vi "Test Serialize.vi"() -> ()   [LabVIEW 2016]
uses:
  typedefs/Request--Cluster.ctl
  JSON-RPC.lvclass
  <vilib>/addons/_JKI.lib/Serialization/JSON/JKI JSON Serialization.lvlib
panel:
  in  "Enum":T1(ring)
  out "x = y?":bool
  in  "Numeric":i32=100 format="%.0p"
  out "x-y":dbl format="%#_6p"
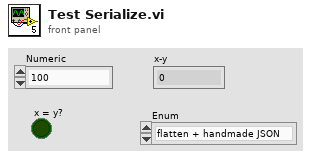
[diagram p1: front panel]
types:
  T1 = enum16{"flatten + handmade JSON", "flatten + JKI JSON", "flatten"}
  T2 = cluster{"jsonrpc":string, "result":string, "error":variant, "id":string}
  T3 = typedef "JSON-RPC.lvclass/Request--Cluster.ctl" = cluster{"method":string, "params":variant, "Notification?":bool}
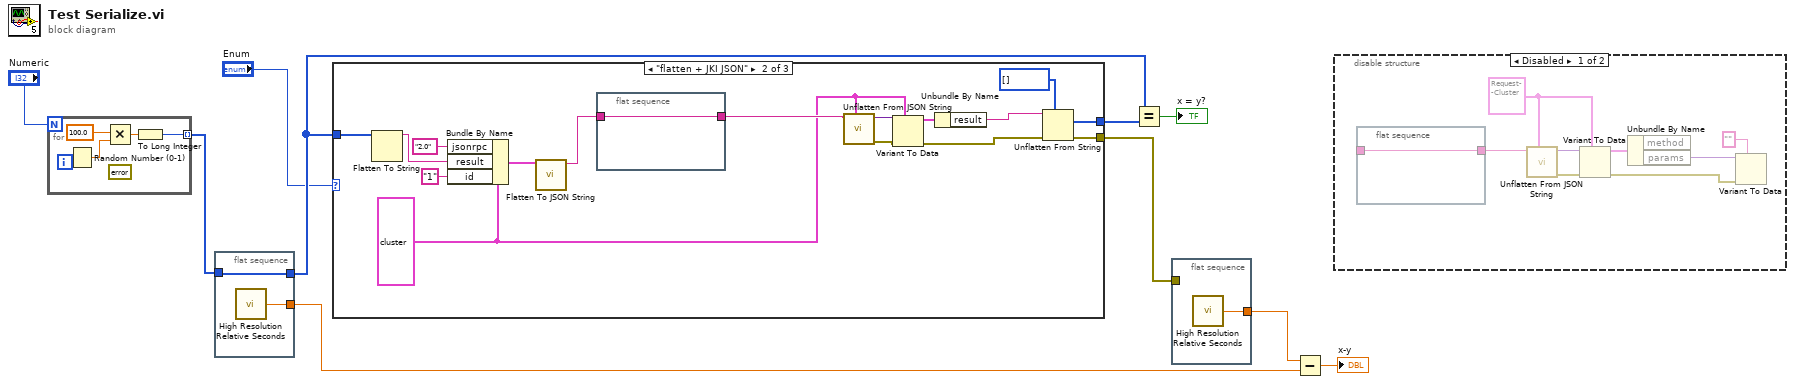
[diagram p0: block diagram]
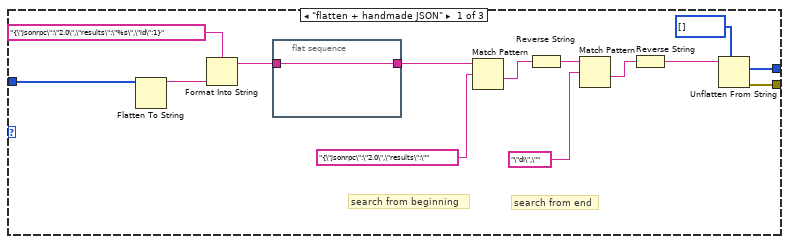
[diagram p2: hidden frame]
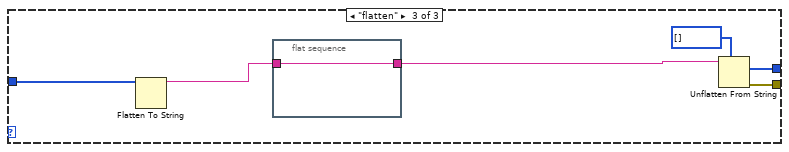
[diagram p3: hidden frame]
diagram:
  n1 = for {
    N: "Numeric" -> [_]
    tunnel: [w11] -> w5 mode=indexing
    (unwired) errorcluster {"status"=FALSE, "code"=0, "source"=""} ("error in (no error)")
    n2 = Random Number (0-1)() -> (number: 0 to 1=w12:dbl)
    n3 = Multiply(x=100.0, y=w12) -> (x*y=w14:dbl)
    n4 = To Long Integer(number=w14) -> (32bit integer=w11:i32)
  }
  n5 = flat-sequence {
    tunnel: [w15] -> w3
    tunnel: [w16] -> w8
    tunnel: w5 -> [w15]
    frame #0 {
      n6 = call <vilib>:"High Resolution Relative Seconds.vi"() -> ("relative seconds"=w16:dbl)
    }
  }
  n7 = case shown="\"flatten + JKI JSON\"" "Enum" {
    tunnel: [w19 w46 w53] -> w6
    tunnel: [w18 w45 w52] -> w4
    tunnel: w3 -> [w17 w44 w51]
    frame "flatten + handmade JSON" {
      # "search from end"
      # "search from beginning"
      n8 = Flatten To String(anything=w17) -> (data string=w30:string)  [unwired: 3 in, 2 out]
      n9 = Format Into String(format string="{\"jsonrpc\":\"2.0\",\"results\":\"%s\",\"id\":1}", w30) -> (resulting string=w27:string)  [unwired: 2 in, 1 out]
      n10 = flat-sequence {
        tunnel: w27 -> [w31]
        tunnel: [w31] -> w26
        frame #0 {
        }
      }
      n11 = Match Pattern(string=w26, regular expression="{\"jsonrpc\":\"2.0\",\"results\":\"") -> (after substring=w25:string)  [unwired: 1 in, 3 out]
      n12 = Reverse String(1:w25) -> (0:w24:string)
      n13 = Match Pattern(string=w24, regular expression="\"di\",\"") -> (after substring=w22:string)  [unwired: 1 in, 3 out]
      n14 = Reverse String(1:w22) -> (0:w21:string)
      n15 = Unflatten From String(type=i32[] [] ("data"), binary string=w21) -> (value=w18:i32[], error out=w19:errorcluster)  [unwired: 3 in, 1 out]
    }
    frame "flatten + JKI JSON" {
      w34 = T2 {"jsonrpc"="", "result"="", "error"=variant, "id"=""} ("response")
      n16 = Flatten To String(anything=w44) -> (data string=w41:string)  [unwired: 3 in, 2 out]
      n17 = Bundle By Name(cluster=w34, "jsonrpc"="2.0", "result"=w41, "id"="1") -> (w40:T2)
      n18 = call <vilib>:"Flatten To JSON String.vi"("Variant"=w40) -> ("JSON String"=w39:string)  [unwired: 9 in, 1 out]
      n19 = flat-sequence {
        tunnel: w39 -> [w48]
        tunnel: [w48] -> w38
        frame #0 {
        }
      }
      n20 = call <vilib>:"Unflatten From JSON String.vi"("Type and Defaults"=w34, "JSON String"=w38) -> ("error out"=w35:errorcluster, "Variant"=w37:variant)  [unwired: 8 in]
      n21 = Variant To Data(error in=w35, type=w34, Variant=w37) -> (data=w36:T2, error out=w32:errorcluster)
      n22 = Unbundle By Name(w36) -> ("result"=w33:string)
      n23 = Unflatten From String(type=i32[] [] ("data"), binary string=w33, error in (no error)=w32) -> (value=w45:i32[], error out=w46:errorcluster)  [unwired: 2 in, 1 out]
    }
    frame "flatten" {
      n24 = Flatten To String(anything=w51) -> (data string=w50:string)  [unwired: 3 in, 2 out]
      n25 = flat-sequence {
        tunnel: w50 -> [w55]
        tunnel: [w55] -> w49
        frame #0 {
        }
      }
      n26 = Unflatten From String(type=i32[] [] ("data"), binary string=w49) -> (value=w52:i32[], error out=w53:errorcluster)  [unwired: 3 in, 1 out]
    }
  }
  n27 = Equal?(x=w3, y=w4) -> (x = y?=→"x = y?":bool)
  n28 = flat-sequence {
    tunnel: [w56] -> w9
    tunnel: w6 -> [_]
    frame #0 {
      n29 = call <vilib>:"High Resolution Relative Seconds.vi"() -> ("relative seconds"=w56:dbl)
    }
  }
  n30 = Subtract(x=w9, y=w8) -> (x-y=→"x-y":dbl)
  n31 = disable-structure shown="Disabled" {
    frame Disabled {
      w62 = T3 {"method"="", "params"=variant, "Notification?"=FALSE} ("request")
      n32 = flat-sequence {
        tunnel: _ -> [w66]
        tunnel: [w66] -> w65
        frame #0 {
        }
      }
      n33 = call <vilib>:"Unflatten From JSON String.vi"("Type and Defaults"=w62, "JSON String"=w65) -> ("error out"=w64:errorcluster, "Variant"=w63:variant, "error in (no error)"=w58:errorcluster)  [unwired: 7 in]
      n34 = Variant To Data(error in=w64, type=w62, Variant=w63) -> (data=w61:T3, error out=w57:errorcluster)
      n35 = Unbundle By Name(w61) -> ("params"=w60:variant)  [unwired: 1 out]
      n36 = Variant To Data(error in=w57, type="", Variant=w60) -> ()  [unwired: 2 out]
    }
    frame Enabled {
    }
  }
